vi "Test_Copy_Array_To_Image_ARGBPixel.vi"(8 "error in (no error)":errorcluster, 11 "Test Case In":refnum<class "Image.lvclass">) -> (0 "error out":errorcluster, 3 "Test Case Out":refnum<class "Image.lvclass">)   [LabVIEW 2020, in "g_ar_toolkit.test.lvlib" / "Image.lvclass"]
uses:
  Image.lvclass
  Image.lvclass/Image.ctl
  g_ar_toolkit.image/g_ar_toolkit.image.lvlib
  g_ar_toolkit.image/Image Size (Fixed).ctl
  g_ar_toolkit.image/CreateEmptyImageARGB.vi
  4993e8ee-a06a-463a-9684-69129f64d5ce.vi
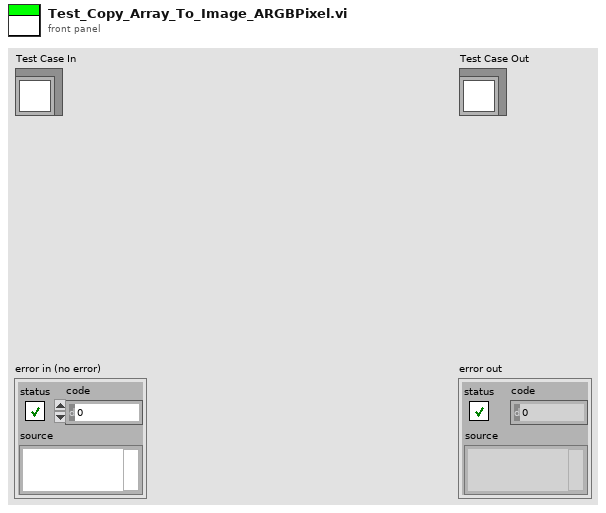
[diagram p1: front panel]
types:
  T1 = typedef "g_ar_toolkit.image.lvlib/Image Size (Fixed).ctl" = cluster{"Width":u16, "Height":u16}
  T2 = typedef "imagedata.ctl" = cluster{"image type":i32, "image depth":i32, "image":u8[], "mask":u8[], "colors":u32[], "Rectangle":cluster{"left":i16, "top":i16, "right":i16, "bottom":i16}}
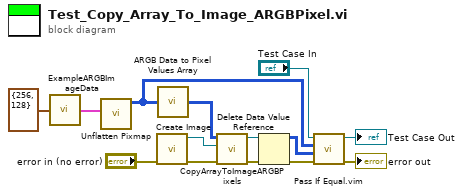
[diagram p0: block diagram]
diagram:
  n1 = call "ExampleARGBImageData.vi"("Image Size"=T1 {"Width"=256, "Height"=128}) -> ("RGB Image Data"=w5:T2)
  n2 = call <vilib>:"Unflatten Pixmap.vi"("image data"=w5) -> ("24-bit pixmap"=w4:u32[][])  [unwired: 4 in, 6 out]
  n3 = call-poly "Create Image.vi"("error in (no error)"="error in (no error)") -> ("error out"=w7:errorcluster, "New ARGB Image"=w6:refnum<data-value>)  [unwired: 9 in]
  n4 = call "ARGB Data to Pixel Values Array.vi"("ARGB Data"=w4) -> ("Pixel Values"=w3:u8[][][])
  n5 = call "CopyArrayToImageARGBPixels.vi"("error in (no error)"=w7, "ARGB Image Destination"=w6, "Source"=w3) -> ("error out"=w2:errorcluster, "ARGB Image Destination (Duplicate)"=w1:refnum<data-value>)  [unwired: 7 in]
  n6 = Delete Data Value Reference(data value reference=w1, error in=w2) -> (data value=w11:u32[][], error out=w9:errorcluster)
  n7 = call "Pass If Equal.vim"("error in (no error)"=w9, "Actual"=w11, "Expected"=w4, "LUnit Test Case In"="Test Case In") -> ("error out"=→"error out":errorcluster, "LUnit Test Case Out"=→"Test Case Out":refnum<class "Image.lvclass">)  [unwired: 6 in]
